vi "Command and Response7265.vi"(8 "error in (no error)":errorcluster, 10 "Command":string="OA.", 11 "7265 GPIB":string="7") -> (0 "error out":errorcluster, 2 "Response Code Only":dbl=0.3, 3 "Response":string="3.0E-01\r\n")   [LabVIEW 2014]
panel:
  out "Response Description":string="\r\n"
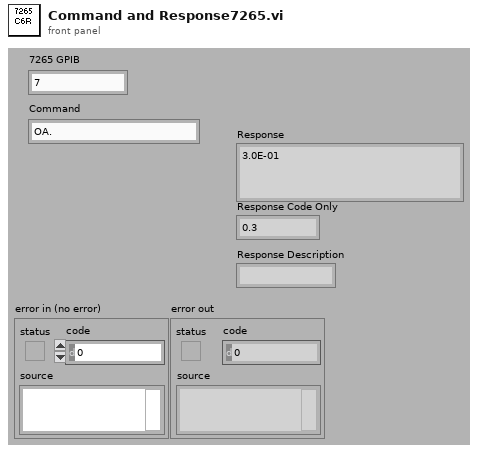
[diagram p1: front panel]
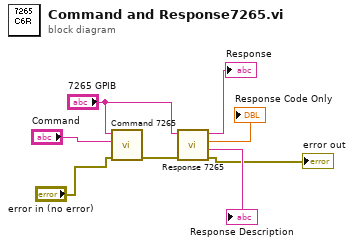
[diagram p0: block diagram]
diagram:
  n1 = call "Command 7265.vi"("error in (no error)"="error in (no error)", "Command"="Command", "7265 GPIB"="7265 GPIB") -> ("error out"=w5:errorcluster)  [unwired: 8 in]
  n2 = call "Response 7265.vi"("error in (no error)"=w5, "7265 GPIB"="7265 GPIB") -> ("error out"=→"error out":errorcluster, "Response Description"=→"Response Description":string, "Response Code Only"=→"Response Code Only":dbl, "Response"=→"Response":string)  [unwired: 6 in]
